vi "Dice.vi"() -> ()   [LabVIEW 2015]
panel:
  in  "Dive Value":bool[](array[boolean])
  in  "Dice":bool
  out "YLDRMErrorOut":errorcluster
  out "YLDRMPortOut":refnum<visa-resource-name>
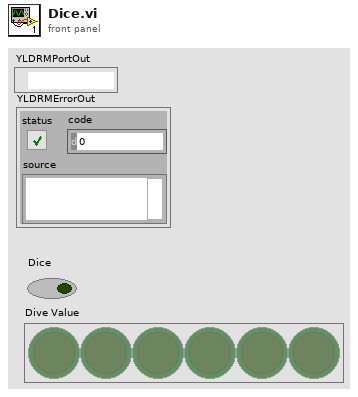
[diagram p1: front panel]
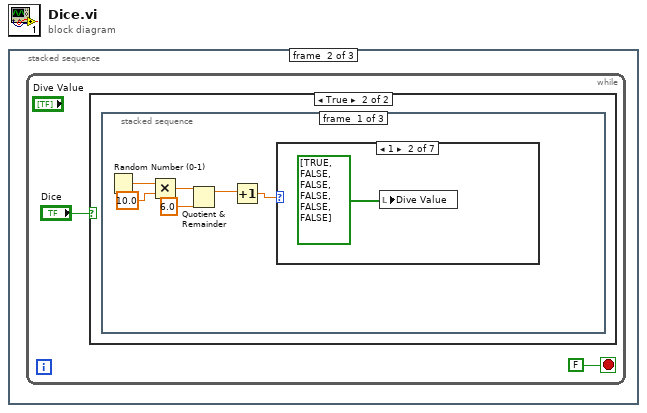
[diagram p0: block diagram]
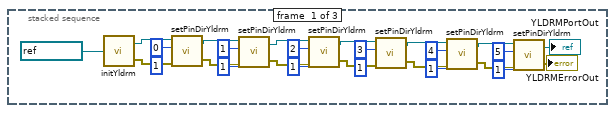
[diagram p2: hidden frame]
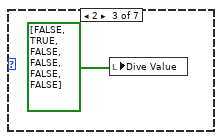
[diagram p5: hidden frame]
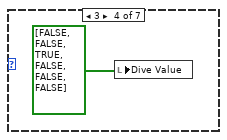
[diagram p6: hidden frame]
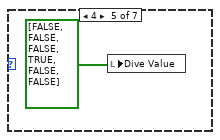
[diagram p7: hidden frame]
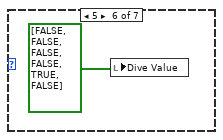
[diagram p8: hidden frame]
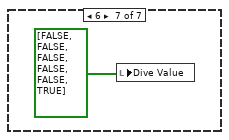
[diagram p9: hidden frame]
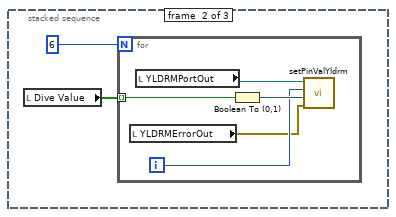
[diagram p10: hidden frame]
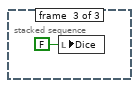
[diagram p11: hidden frame]
diagram:
  n1 = stacked-sequence {
    frame #0 {
      n2 = call "initYldrm.vi"("YLDRMPortInp"=refnum<visa-resource-name> "COM9") -> ("YLDRMPortOut"=w26:refnum<visa-resource-name>, "YLDRMErrorOut"=w25:errorcluster)
      n3 = call "setPinDirYldrm.vi"("YLDRMErrorInp"=w25, "dir"=u8 1, "pin"=u8 0, "YLDRMPortInp"=w26) -> ("YLDRMErrorOut"=w19:errorcluster, "YLDRMPortOut"=w20:refnum<visa-resource-name>)
      n4 = call "setPinDirYldrm.vi"("YLDRMErrorInp"=w19, "dir"=u8 1, "pin"=u8 1, "YLDRMPortInp"=w20) -> ("YLDRMErrorOut"=w11:errorcluster, "YLDRMPortOut"=w12:refnum<visa-resource-name>)
      n5 = call "setPinDirYldrm.vi"("YLDRMErrorInp"=w11, "dir"=u8 1, "pin"=u8 2, "YLDRMPortInp"=w12) -> ("YLDRMErrorOut"=w18:errorcluster, "YLDRMPortOut"=w17:refnum<visa-resource-name>)
      n6 = call "setPinDirYldrm.vi"("YLDRMErrorInp"=w18, "dir"=u8 1, "pin"=u8 3, "YLDRMPortInp"=w17) -> ("YLDRMErrorOut"=w3:errorcluster, "YLDRMPortOut"=w4:refnum<visa-resource-name>)
      n7 = call "setPinDirYldrm.vi"("YLDRMErrorInp"=w3, "dir"=u8 1, "pin"=u8 4, "YLDRMPortInp"=w4) -> ("YLDRMErrorOut"=w5:errorcluster, "YLDRMPortOut"=w6:refnum<visa-resource-name>)
      n8 = call "setPinDirYldrm.vi"("YLDRMErrorInp"=w5, "dir"=u8 1, "pin"=u8 5, "YLDRMPortInp"=w6) -> ("YLDRMErrorOut"=→"YLDRMErrorOut":errorcluster, "YLDRMPortOut"=→"YLDRMPortOut":refnum<visa-resource-name>)
    }
    frame #1 {
      n9 = while {
        stop <- FALSE stop-if-true
        n10 = case shown="True" "Dice" {
          frame False {
          }
          frame True {
            n11 = stacked-sequence {
              frame #0 {
                n12 = Random Number (0-1)() -> (number: 0 to 1=w35:dbl)
                n13 = Multiply(x=w35, y=10.0) -> (x*y=w33:dbl)
                n14 = Quotient & Remainder(x=w33, y=6.0) -> (x-y*floor(x/y)=w31:dbl)  [unwired: 1 out]
                n15 = Increment(x=w31) -> (x+1=w30:dbl)
                n16 = case shown="1" w30 {
                  frame 0, Default {
                  }
                  frame 1 {
                    n17 = local write "Dive Value"(bool[] [TRUE, FALSE, FALSE, FALSE, FALSE, FALSE] ("Dive Value")) -> ()
                  }
                  frame 2 {
                    n18 = local write "Dive Value"(bool[] [FALSE, TRUE, FALSE, FALSE, FALSE, FALSE] ("Dive Value")) -> ()
                  }
                  frame 3 {
                    n19 = local write "Dive Value"(bool[] [FALSE, FALSE, TRUE, FALSE, FALSE, FALSE] ("Dive Value")) -> ()
                  }
                  frame 4 {
                    n20 = local write "Dive Value"(bool[] [FALSE, FALSE, FALSE, TRUE, FALSE, FALSE] ("Dive Value")) -> ()
                  }
                  frame 5 {
                    n21 = local write "Dive Value"(bool[] [FALSE, FALSE, FALSE, FALSE, TRUE, FALSE] ("Dive Value")) -> ()
                  }
                  frame 6 {
                    n22 = local write "Dive Value"(bool[] [FALSE, FALSE, FALSE, FALSE, FALSE, TRUE] ("Dive Value")) -> ()
                  }
                }
              }
              frame #1 {
                n23 = local read "Dive Value"() -> (w42:bool[])
                n24 = for {
                  N: 6 -> [_]
                  tunnel: w42 -> [w48] mode=indexing
                  i -> [w46]
                  n25 = local read "YLDRMErrorOut"() -> (w45:errorcluster)
                  n26 = local read "YLDRMPortOut"() -> (w44:refnum<visa-resource-name>)
                  n27 = Boolean To (0,1)(Boolean=w48) -> (0, 1=w47:i16)
                  n28 = call "setPinValYldrm.vi"("YLDRMErrorInp"=w45, "val"=w47, "pin"=w46, "YLDRMPortInp"=w44) -> ()  [unwired: 2 out]
                }
              }
              frame #2 {
                n29 = local write "Dice"(FALSE ("Dice")) -> ()
              }
            }
          }
        }
      }
    }
    frame #2 {
    }
  }
